vi "Controller Diagnostics Data.vi"() -> ()   [LabVIEW 2011, in "Controller Global Variables.lvlib"]
uses:
  Controller Global Variables.lvlib
  Types Definitions/Type Diagnostics Data.ctl
  Types Definitions/Type CPU Loads Array.ctl
  Types Definitions/Type CPU Loads.ctl
  Type Definitions.lvlib
panel:
  in  "Diagnostics Data":T1 {"CPU Loads Array"."ISR (%)" format="%#.2f"; "CPU Loads Array"."Idle (%)" format="%#.2f"; "CPU Loads Array"."Background (%)" format="%#.2f"; "CPU Loads Array"."Normal (%)" format="%#.2f"; "CPU Loads Array"."Above Normal (%)" format="%#.2f"; "CPU Loads Array"."High (%)" format="%#.2f"; "CPU Loads Array"."Timed Structures (%)" format="%#.2f"; "CPU Loads Array"."Time Critical (%)" format="%#.2f"; "CPU Loads Array"."Total (%)" format="%#.2f"}
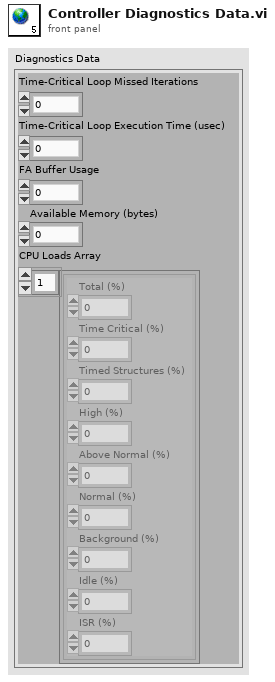
[diagram p1: front panel]
types:
  T1 = typedef "Type Definitions.lvlib/Type Diagnostics Data.ctl" = cluster{"Time-Critical Loop Missed Iterations":u32, "Time-Critical Loop Execution Time (usec)":u32, "FA Buffer Usage":u32, "Available Memory (bytes)":u32, "CPU Loads Array":T2}
  T2 = typedef "Type Definitions.lvlib/Type CPU Loads Array.ctl" = T3[]
  T3 = typedef "Type Definitions.lvlib/Type CPU Loads.ctl" = cluster{"Total (%)":dbl, "Time Critical (%)":dbl, "Timed Structures (%)":dbl, "High (%)":dbl, "Above Normal (%)":dbl, "Normal (%)":dbl, "Background (%)":dbl, "Idle (%)":dbl, "ISR (%)":dbl}
diagram:
